vi "Measurements Operations_Meas-Scope SP.vi"(7 "Opearte":T3=enum."Config&Read", 8 "error in":errorcluster, 9 "Config":T2, 10 "Index":i32, 11 "InstruHandle":refnum<k15>) -> (0 "error out":errorcluster, 1 "ConfigOut":T1(array[cluster]), 2 "Items":string[][](array[string]), 3 "Results":string[](array[string]))   [LabVIEW 2012]
uses:
  Measure Operations_Meas.ctl
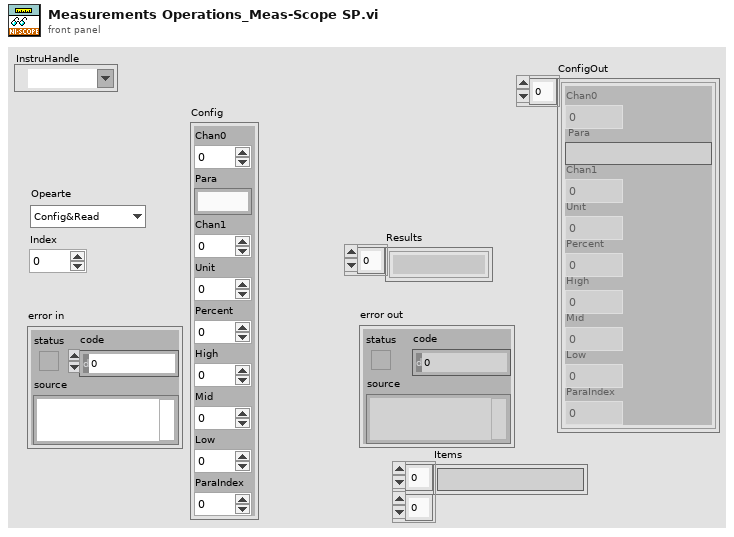
[diagram p1: front panel]
types:
  T1 = cluster{"Chan0":i32, "Para":string, "Chan1":i32, "Unit":i32, "Percent":i32, "High":dbl, "Mid":dbl, "Low":dbl, "ParaIndex":i32}[]
  T2 = cluster{"Chan0":i32, "Para":string, "Chan1":i32, "Unit":i32, "Percent":i32, "High":dbl, "Mid":dbl, "Low":dbl, "ParaIndex":i32}
  T3 = typedef "Measure Operations_Meas.ctl" = enum16{"Add", "Config&Read", "Delete", "Clear"}
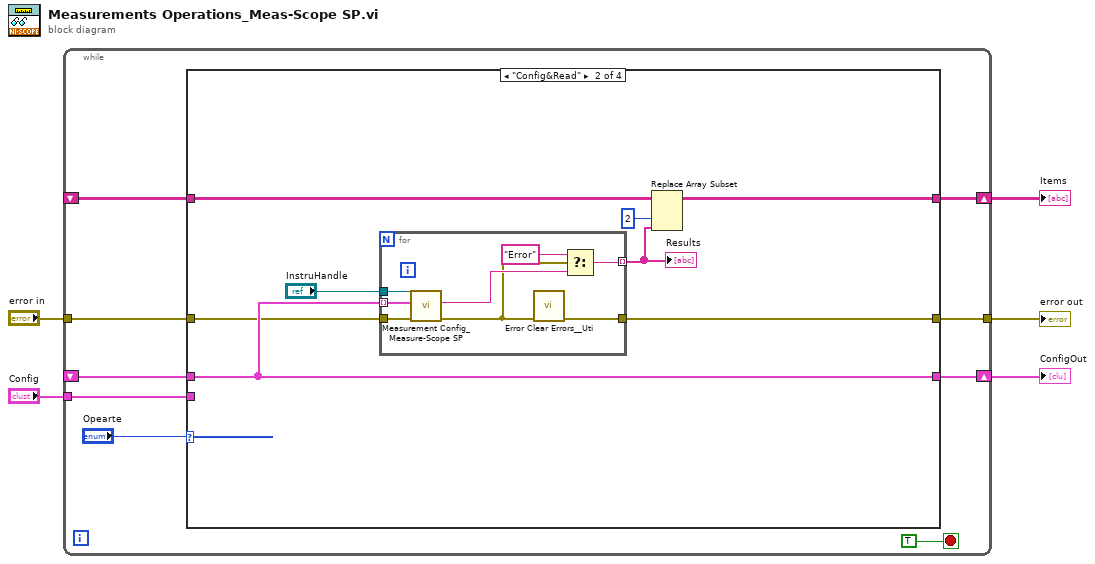
[diagram p0: block diagram]
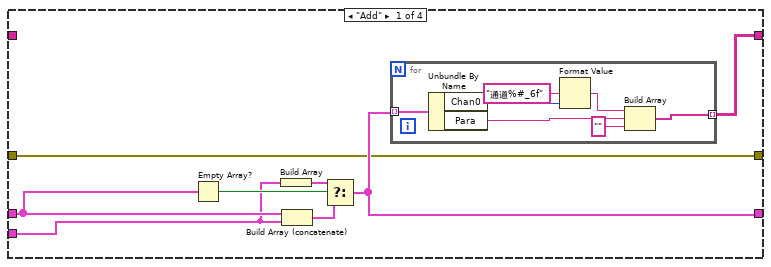
[diagram p2: hidden frame]
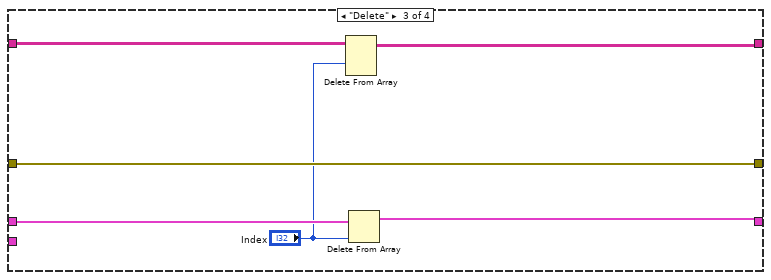
[diagram p3: hidden frame]
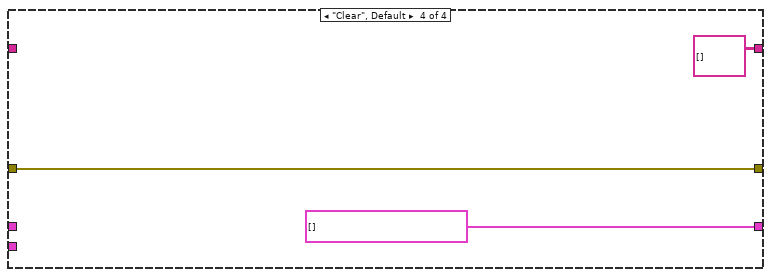
[diagram p4: hidden frame]
diagram:
  n1 = while {
    shift-right: [w12] -> w2
    shift-left: _ -> [w11]
    tunnel: "error in" -> [w6]
    tunnel: "Config" -> [w10]
    tunnel: [w9] -> w3
    shift-right: [w8] -> w1
    shift-left: _ -> [w7]
    stop <- TRUE stop-if-true
    n2 = case shown="\"Config&Read\"" "Opearte" {
      tunnel: [w19 w36 w49 T1 [] ("Config")] -> w12
      tunnel: w11 -> [w21 w36 w50 _]
      tunnel: w6 -> [w17 w33 w51 w53]
      tunnel: w10 -> [w18 _ _ _]
      tunnel: [w17 w37 w51 w53] -> w9
      tunnel: [w22 w34 w46 string[][] []] -> w8
      tunnel: w7 -> [_ w35 w48 _]
      frame "Add" {
        n3 = Empty Array?(array=w21) -> (empty?=w20:bool)
        n4 = Build Array(w18) -> (w16:T1)
        n5 = Build Array (concatenate)(w21, w18) -> (w15:T1)
        n6 = Select(t=w16, s=w20, f=w15) -> (s? t:f=w19:T1)
        n7 = for {
          tunnel: w19 -> [w29] mode=indexing
          tunnel: [w24] -> w22 mode=indexing
          n8 = Unbundle By Name(w29) -> ("Chan0"=w28:i32, "Para"=w25:string)
          n9 = Format Value(format string="通道%#_6f", value (0)=w28) -> (output string=w26:string)  [unwired: 1 in]
          n10 = Build Array(w26, w25, "") -> (w24:string[])
        }
      }
      frame "Config&Read" {
        n11 = for {
          tunnel: w36 -> [w44] mode=indexing
          tunnel: w33 -> [w45]
          tunnel: [w39] -> w37
          tunnel: [w41] -> w31 mode=indexing
          tunnel: "InstruHandle" -> [w38]
          n12 = call "Measurement Config_Measure-Scope SP.vi"("error in"=w45, "Config"=w44, "InstruHandle"=w38) -> ("error out"=w40:errorcluster, "Result"=w42:string)  [unwired: 7 in]
          n13 = call "Error Clear Errors__Uti.vi"("error in (no error)"=w40) -> ("error out"=w39:errorcluster)  [unwired: 6 in]
          n14 = Select(t="Error", s=w40, f=w42) -> (s? t:f=w41:string)
        }
        "Results" <- w31
        n15 = Replace Array Subset(array=w35, new element=w31, index (col)=2 ("disabled index (col)")) -> (w34:string[][])  [unwired: 1 in]
      }
      frame "Delete" {
        n16 = Delete From Array(array=w48, index (row)="Index") -> (array with subset deleted=w46:string[][])  [unwired: 2 in, 1 out]
        n17 = Delete From Array(array=w50, index="Index") -> (array with subset deleted=w49:T1)  [unwired: 1 in, 1 out]
      }
      frame "Clear", Default {
      }
    }
  }
  "error out" <- w3
  "ConfigOut" <- w2
  "Items" <- w1
